vi "Unified Msgs.vi"(6 "Alias":string, 7 "Actor in":refnum<class "Actor.lvclass">) -> (0 "Error out":errorcluster, 2 "Unified Msgs":T1)   [LabVIEW 2020, in "jettl.lvlib" / "Read Child Attributes.lvlib"]
uses:
  Read Child Attributes.lvlib
  jettl.lvlib
  Attributes/Attributes.lvclass
  Actor/Actor.lvclass
  Msg/Msg.lvclass
  Msgs.ctl
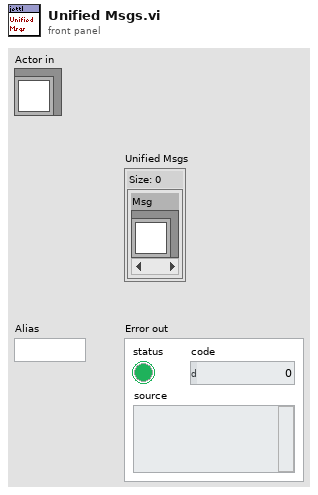
[diagram p1: front panel]
types:
  T1 = typedef "jettl.lvlib/Msgs.ctl" = set{refnum<class "Msg.lvclass">}
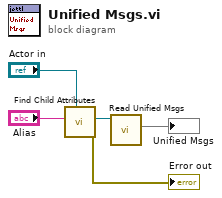
[diagram p0: block diagram]
diagram:
  n1 = call "Find Child Attributes.vi"("Actor in"="Actor in", "Alias"="Alias") -> ("Error out"=→"Error out":errorcluster, "Child Attributes"=w2:refnum<class "Attributes.lvclass">)  [unwired: 8 in]
  n2 = call-dynamic "Read Unified Msgs.vi"("Attributes in"=w2) -> ("Unified Msgs"=→"Unified Msgs":T1)  [unwired: 10 in]
